vi "Read ConvBox Handler.vi"(8 "error in (no error)":errorcluster, 11 "Listener in":refnum<class "Listener.lvclass">) -> (0 "error out":errorcluster, 3 "Listener out":refnum<class "Listener.lvclass">)   [LabVIEW 2023, in "Listener.lvclass"]
uses:
  Listener.lvclass
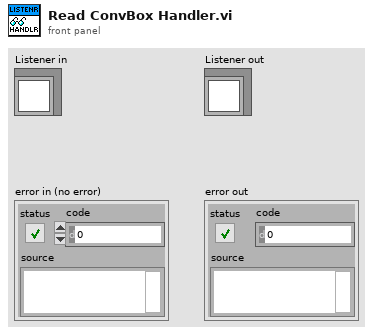
[diagram p1: front panel]
types:
  T1 = typedef "Listener.lvclass/RS-xxx To GPIB ConvBox Data Structure.ctl" = cluster{"Data":string, "Command Messages Read":string[], "Address":string, "Data Length":u32}
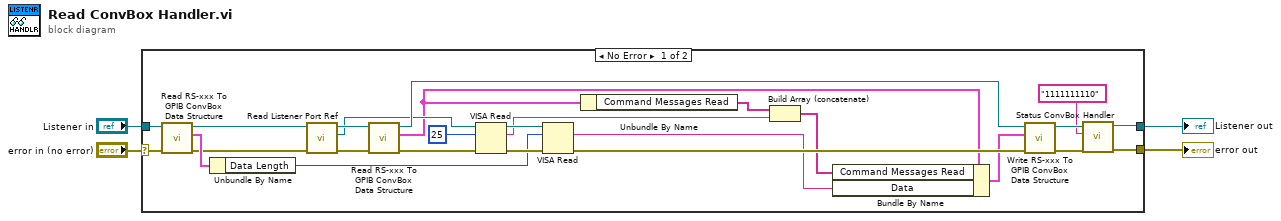
[diagram p0: block diagram]
diagram:
  n1 = case shown="No Error" "error in (no error)" {
    selector: "error in (no error)" -> [w15 w31]
    tunnel: "Listener in" -> [w16 w32]
    tunnel: [w23 w31] -> w2
    tunnel: [w22 w32] -> w1
    frame No Error {
      n2 = call-dynamic "Read RS-xxx To GPIB ConvBox Data Structure.vi"("error in (no error)"=w15, "Listener in"=w16) -> ("error out"=w13:errorcluster, "RS-xxx To GPIB ConvBox Data Structure"=w14:T1, "Listener out"=w12:refnum<class "Listener.lvclass">)  [unwired: 7 in]
      n3 = Unbundle By Name(w14) -> ("Data Length"=w11:u32)
      n4 = call "Read Listener Port Ref.vi"("error in (no error)"=w13, "Listener in"=w12) -> ("error out"=w19:errorcluster, "Listener Port Ref"=w18:refnum<visa-resource-name>, "Listener out"=w20:refnum<class "Listener.lvclass">)  [unwired: 7 in]
      n5 = call-dynamic "Read RS-xxx To GPIB ConvBox Data Structure.vi"("error in (no error)"=w19, "Listener in"=w20) -> ("error out"=w21:errorcluster, "RS-xxx To GPIB ConvBox Data Structure"=w8:T1, "Listener out"=w25:refnum<class "Listener.lvclass">)  [unwired: 7 in]
      n6 = VISA Read(VISA resource name=w18, byte count=u32 25, error in (no error)=w21) -> (VISA resource name out=w30:refnum<visa-resource-name>, read buffer=w9:string, error out=w29:errorcluster)  [unwired: 1 out]
      n7 = VISA Read(VISA resource name=w30, byte count=w11, error in (no error)=w29) -> (read buffer=w6:string, error out=w27:errorcluster)  [unwired: 2 out]
      n8 = Unbundle By Name(w8) -> ("Command Messages Read"=w10:string[])
      n9 = Build Array (concatenate)(w10, w9) -> (w7:string[])
      n10 = Bundle By Name(cluster=w8, "Command Messages Read"=w7, "Data"=w6) -> (w5:T1)
      n11 = call-dynamic "Write RS-xxx To GPIB ConvBox Data Structure.vi"("error in (no error)"=w27, "RS-xxx To GPIB ConvBox Data Structure"=w5, "Listener in"=w25) -> ("error out"=w26:errorcluster, "Listener out"=w24:refnum<class "Listener.lvclass">)  [unwired: 7 in]
      n12 = call "Status ConvBox Handler.vi"("error in(no error)"=w26, "Value In"="1111111110" ("write buffer"), "Listener in"=w24) -> ("error out"=w23:errorcluster, "Listener out"=w22:refnum<class "Listener.lvclass">)  [unwired: 7 in]
    }
    frame Error {
    }
  }
  "error out" <- w2
  "Listener out" <- w1
